vi "Detect Guilty Packages.vi"() -> ()   [LabVIEW 2019]
uses:
  Build/Project.Dependencies Finder.lvlibp/1abvi3w/vi.lib/Utility/sysdir.llb/Project.Dependencies Finder_System Directory Type.ctl
  Build/Project.Dependencies Finder.lvlibp
  Build/Project.Dependencies Finder.lvlibp/Dependency Source_VIPM/Dependency Source_VIPM.lvclass
panel:
  out "error out":errorcluster
  in  "search string":string="openg"
  out "Package list that contains search string":string[](array[string])
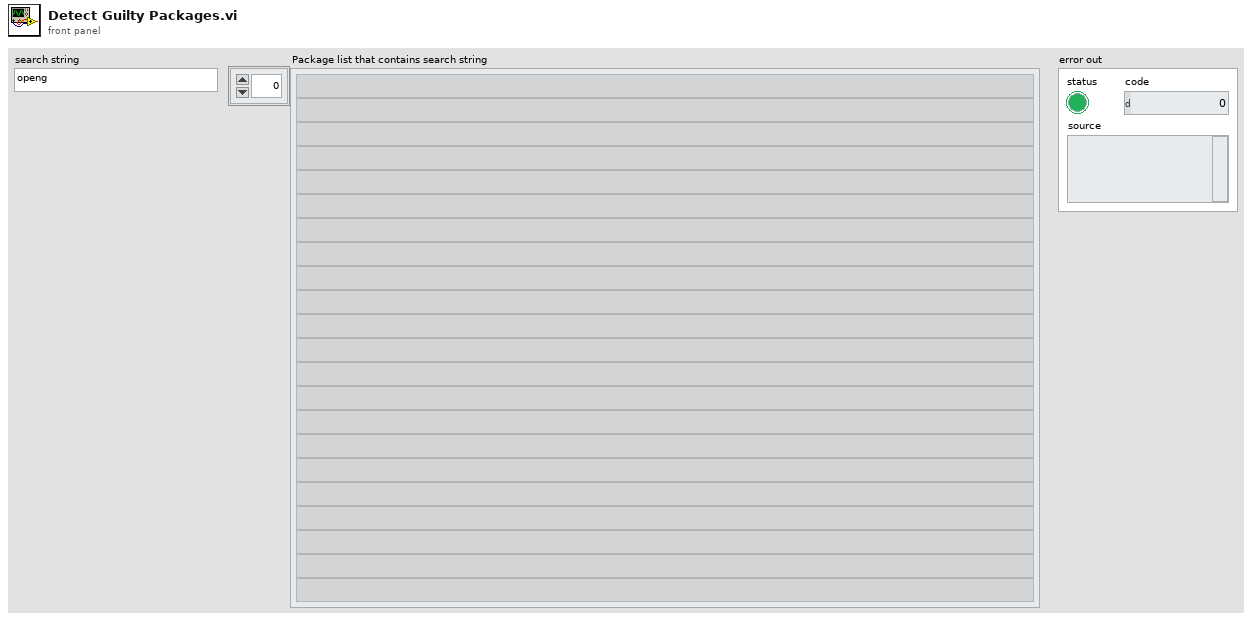
[diagram p1: front panel]
types:
  T1 = typedef "Project.Dependencies Finder.lvlibp/Project.Dependencies Finder_System Directory Type.ctl" = i32
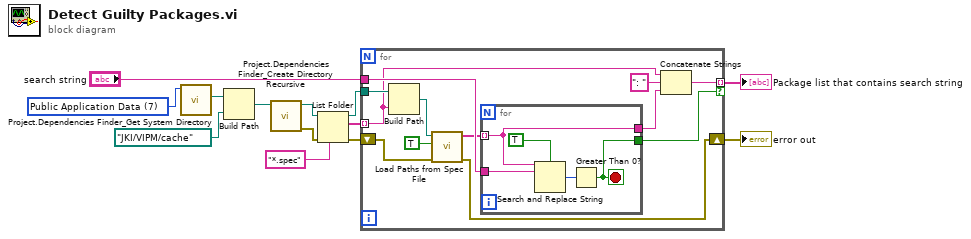
[diagram p0: block diagram]
diagram:
  w7 = T1 7 items=["User Home"=0, "User Desktop"=1, "User Documents"=2, "User Application Data"=3, "User Preferences"=4, "User Temporary"=5, "Public Documents"=6, "Public Application Data"=7, "Public Preferences"=8, "Public Cache"=13, "System Core Libraries"=9, "System Installed Libraries"=10, "Application Files"=11, "Boot Volume Root"=12] ("system directory type")
  n1 = call "Project.Dependencies Finder_Get System Directory.vi"("system directory type"=w7) -> ("system directory"=w8:path)  [unwired: 10 in]
  n2 = Build Path(base path=w8, name or relative path=path "JKI/VIPM/cache") -> (appended path=w9:path)
  n3 = call "Project.Dependencies Finder_Create Directory Recursive.vi"("directory"=w9) -> ("error out"=w5:errorcluster, "directory copy"=w13:path)  [unwired: 4 in, 1 out]
  n4 = List Folder(path=w13, pattern="*.spec", error in=w5) -> (path out=w6:path, filenames=w12:string[], error out=w2:errorcluster)  [unwired: 1 in, 1 out]
  n5 = for {
    tunnel: w6 -> [w25]
    tunnel: w12 -> [w19] mode=indexing
    tunnel: "search string" -> [w22]
    tunnel: [w17] -> w3 mode=indexing if=w16
    shift-right: [w14] -> w1
    shift-left: w2 -> [w15]
    n6 = Build Path(base path=w25, name or relative path=w19) -> (appended path=w24:path)
    n7 = call "Load Paths from Spec File.vi"("error in (no error)"=w15, "Highest Version?"=TRUE, "Spec path"=w24) -> ("error out"=w14:errorcluster, "External Path Combinations"=w18:string[])  [unwired: 6 in, 1 out]
    n8 = for {
      tunnel: w18 -> [w26] mode=indexing
      tunnel: [w28] -> w16
      tunnel: w22 -> [w27]
      tunnel: [w26] -> w20
      stop <- w28 stop-if-true
      n9 = Search and Replace String(case sensitive?=TRUE ("ignore case? (F)"), input string=w26, search string=w27) -> (number of replacements=w29:i32)  [unwired: 5 in, 3 out]
      n10 = Greater Than 0?(x=w29) -> (x > 0?=w28:bool)
    }
    n11 = Concatenate Strings(w19, ": " ("string"), w20) -> (w17:string)
  }
  "Package list that contains search string" <- w3
  "error out" <- w1
